vi "cumplimiento.vi"(8 "error in (no error)":errorcluster, 11 "Prueba08 in":refnum<class "Prueba33.lvclass">) -> (0 "error out":errorcluster, 2 "cumpimiento":string, 3 "Prueba08 out":refnum<class "Prueba33.lvclass">)   [LabVIEW 2019, in "Prueba33.lvclass"]
uses:
  Prueba33.lvclass
  Prueba33.lvclass/Prueba33.ctl
  RerenceAllControlsToolkit/_get control reference by name.vi
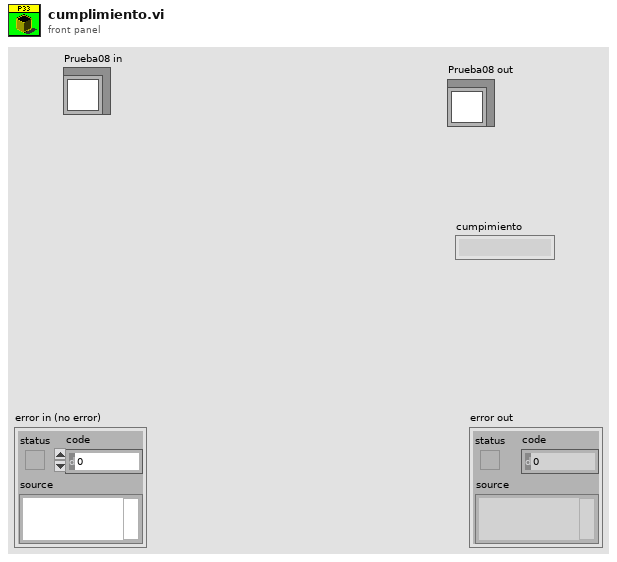
[diagram p1: front panel]
types:
  T1 = cluster{"Medido":dbl, "Error":dbl, "Ref":dbl, "Incert_exp":dbl, "Tol+":dbl, "Tol-":dbl, "fila":i32}
  T2 = cluster{"ControlName":string, "ControlReference":refnum<vi>}[]
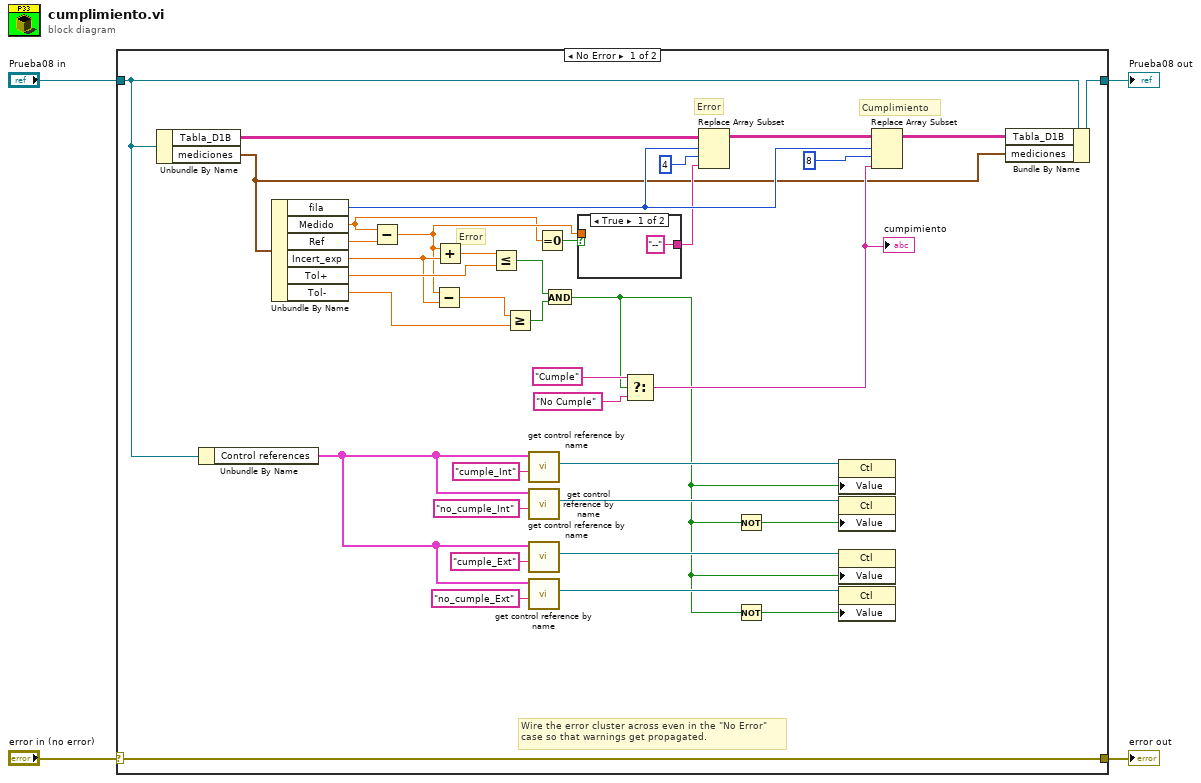
[diagram p0: block diagram]
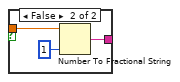
[diagram p2: hidden frame]
diagram:
  n1 = case shown="No Error" "error in (no error)" {
    selector: "error in (no error)" -> [w41 w47]
    tunnel: [w41 w47] -> w3
    tunnel: [w21 w46] -> w2
    tunnel: "Prueba08 in" -> [w17 w46]
    frame No Error {
      # "Cumplimiento"
      # "Error"
      # "Error"
      # "Wire the error cluster across even in the \"No Error\"\ncase so that warnings get propagated."
      n2 = Unbundle By Name(w17) -> ("Tabla_D1B"=w19:string[][], "mediciones"=w18:T1)
      n3 = Unbundle By Name(w17) -> ("Control references"=w6:T2)
      n4 = Unbundle By Name(w18) -> ("fila"=w27:i32, "Medido"=w22:dbl, "Ref"=w34:dbl, "Incert_exp"=w32:dbl, "Tol+"=w33:dbl, "Tol-"=w31:dbl)
      n5 = Subtract(x=w22, y=w34) -> (x-y=w23:dbl)
      n6 = Subtract(x=w23, y=w32) -> (x-y=w37:dbl)
      n7 = Add(x=w23, y=w32) -> (x+y=w40:dbl)
      n8 = Less Or Equal?(x=w40, y=w33) -> (x <= y?=w39:bool)
      n9 = Greater Or Equal?(x=w37, y=w31) -> (x >= y?=w38:bool)
      n10 = call-poly "get control reference by name.vi"("Control name"="cumple_Int", "Control references"=w6) -> ("Ctl Refnum"=w16:refnum<vi>)  [unwired: 4 in, 1 out]
      n11 = call-poly "get control reference by name.vi"("Control name"="no_cumple_Int", "Control references"=w6) -> ("Ctl Refnum"=w13:refnum<vi>)  [unwired: 4 in, 1 out]
      n12 = call-poly "get control reference by name.vi"("Control name"="cumple_Ext", "Control references"=w6) -> ("Ctl Refnum"=w7:refnum<vi>)  [unwired: 4 in, 1 out]
      n13 = call-poly "get control reference by name.vi"("Control name"="no_cumple_Ext", "Control references"=w6) -> ("Ctl Refnum"=w10:refnum<vi>)  [unwired: 4 in, 1 out]
      n14 = Equal To 0?(x=w22) -> (x = 0?=w24:bool)
      n15 = And(x=w39, y=w38) -> (x .and. y?=w5:bool)
      n16 = case shown="True" w24 {
        tunnel: w23 -> [_ w45]
        tunnel: ["--" w43] -> w25
        frame True {
        }
        frame False {
          n17 = Number To Fractional String(number=w45, precision (6)=i16 1) -> (F-format string=w43:string)  [unwired: 2 in]
        }
      }
      n18 = Select(t="Cumple", s=w5, f="No Cumple") -> (s? t:f=w30:string)
      "cumpimiento" <- w30
      n19 = Replace Array Subset(array=w19, new element=w25, index (row)=w27, index (col)=4 ("disabled index (col)")) -> (w28:string[][])
      n20 = Not(x=w5) -> (.not. x?=w12:bool)
      n21 = Not(x=w5) -> (.not. x?=w11:bool)
      n22 = property class="Ctl"(reference=w16, "Value"=w5) -> ()  [unwired: 1 in, 2 out]
      n23 = property class="Ctl"(reference=w13, "Value"=w12) -> ()  [unwired: 1 in, 2 out]
      n24 = property class="Ctl"(reference=w7, "Value"=w5) -> ()  [unwired: 1 in, 2 out]
      n25 = property class="Ctl"(reference=w10, "Value"=w11) -> ()  [unwired: 1 in, 2 out]
      n26 = Replace Array Subset(array=w28, new element=w30, index (row)=w27, index (col)=8 ("index (row)")) -> (w20:string[][])
      n27 = Bundle By Name(cluster=w17, "Tabla_D1B"=w20, "mediciones"=w18) -> (w21:refnum<class "Prueba33.lvclass">)
    }
    frame Error {
    }
  }
  "error out" <- w3
  "Prueba08 out" <- w2
